vi "Calibration.vi"(0 "Enable":bool, 1 "IP.":string caption="IP地址") -> ()   [LabVIEW 2012]
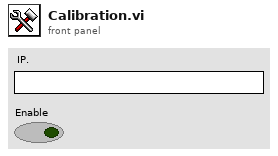
[diagram p1: front panel]
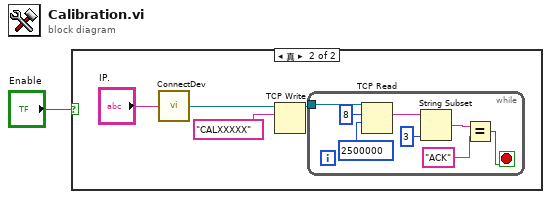
[diagram p0: block diagram]
diagram:
  n1 = case shown="真" "Enable" {
    frame False {
    }
    frame True {
      n2 = call "ConnectDev.vi"("IP."="IP.") -> ("connection ID"=w2:refnum<k5>)
      n3 = TCP Write(connection ID=w2, data in="CALXXXXX" ("数据输入")) -> (connection ID out=w5:refnum<k5>)  [unwired: 2 in, 2 out]
      n4 = while {
        tunnel: w5 -> [w13]
        stop <- w8 stop-if-true
        n5 = TCP Read(connection ID=w13, bytes to read=8 ("读取的字节"), 9:2500000 ("超时毫秒(25000)")) -> (data out=w11:string)  [unwired: 2 in, 2 out]
        n6 = String Subset(string=w11, length (rest)=3 ("偏移量(0)")) -> (substring=w10:string)  [unwired: 1 in]
        n7 = Equal?(x=w10, y="ACK") -> (x = y?=w8:bool)
      }
    }
  }
